vi "Read Analogue.vi"(8 "error in (no error)":errorcluster, 11 "Sim DMM in":refnum<class "Sim DMM.lvclass">) -> (0 "error out":errorcluster, 2 "Waveforms":waveform(dbl)[](array[waveform]), 3 "Sim DMM out":refnum<class "Sim DMM.lvclass">)   [LabVIEW 2025, in "DMM.lvlib" / "Sim DMM.lvclass"]
uses:
  Sim DMM.lvclass
  C:/Users/Public/Documents/Sandia National Labs/TSS Plugin/CEF.lvlibp/Node/CEF_Node.lvclass
  C:/Users/Public/Documents/Sandia National Labs/TSS Plugin/Abstract Engine.lvlibp/Abstract Instrument/Abstract Instrument.lvclass
  Users/Public/Documents/Sandia National Labs/TSS Plugin/Abstract Engine.lvlibp/Abstract Instrument/Channel.ctl
  DMM Channel/DMM Channel.lvclass
  Users/Public/Documents/Sandia National Labs/TSS Plugin/Abstract Engine.lvlibp/Channel configuration/Channel configuration.lvclass
  Users/Public/Documents/Sandia National Labs/TSS Plugin/CEF.lvlibp/Node/ReadChildren.vi
  Users/Public/Documents/Sandia National Labs/TSS Plugin/Abstract Engine.lvlibp/Channel configuration/Read Channel Setting.vi
  Users/Public/Documents/Sandia National Labs/TSS Plugin/CEF.lvlibp/Node/CEF_Node.lvclass
  Users/Public/Documents/Sandia National Labs/TSS Plugin/CEF.lvlibp/serializable configuration/CEF_serializable configuration.lvclass
  <vilib>/ptbypt/NI_PtbyPt.lvlib
  Users/Public/Documents/Sandia National Labs/TSS Plugin/Abstract Engine.lvlibp/Abstract Instrument/Abstract Instrument.lvclass
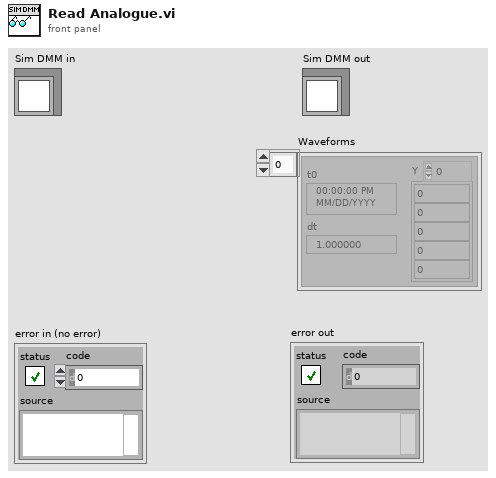
[diagram p1: front panel]
types:
  T1 = typedef "Abstract Engine.lvlibp/Abstract Instrument.lvclass/Channel.ctl" = cluster{"Alias":string, "DataType":enum16{"Anaolg Input", "Waveform"}, "Unit":enum16{"---", "V", "A", "Ohm", "Hz", "uF", "degC", "deg"}, "Upper limit":dbl, "Lower limit":dbl, "Measurement":variant}
  T2 = typedef "Abstract Engine.lvlibp/Channel configuration.lvclass/Default Channel.ctl" = cluster{"Address":string, "SW Alias":string, "Enabled":bool, "Type":string, "Description":string}
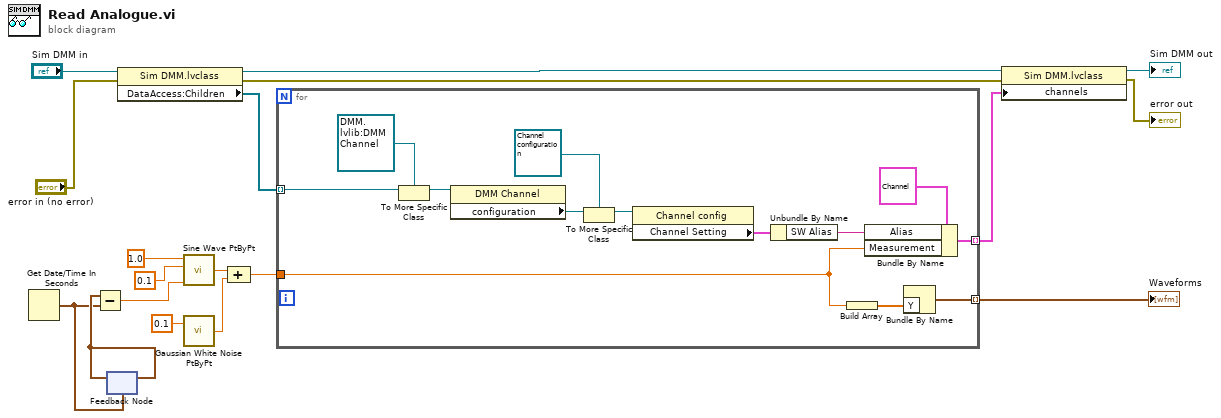
[diagram p0: block diagram]
diagram:
  n1 = Get Date/Time In Seconds() -> (seconds since 1Jan1904=w11:timestamp)
  n2 = feedback #1(w11) -> (w15:timestamp)
  n3 = Subtract(x=w15, y=w11) -> (x-y=w12:dbl)
  n4 = feedback-in #1(w15) -> ()
  n5 = property class="Sim DMM.lvclass"(reference="Sim DMM in", error in="error in (no error)") -> (reference out=w9:refnum<class "Sim DMM.lvclass">, error out=w4:errorcluster, "DataAccess:Children"=w8:refnum<data-value>[])
  n6 = call <vilib>:"Sine Wave PtByPt.vi"("time"=w12, "frequency"=0.1, "amplitude"=1.0) -> ("sine wave"=w17:dbl)  [unwired: 1 in]
  n7 = call <vilib>:"Gaussian White Noise PtByPt.vi"("standard deviation"=0.1) -> ("Gaussian white noise"=w16:dbl)  [unwired: 2 in]
  n8 = Compound Arithmetic op=ADD(w17, w16) -> (w7:dbl)
  n9 = for {
    tunnel: w8 -> [w31] mode=indexing
    tunnel: [w29] -> w2 mode=indexing
    tunnel: w7 -> [w27]
    tunnel: [w25] -> w1 mode=indexing
    n10 = To More Specific Class(target class=refnum<data-value> refnum ("data value reference"), reference=w31) -> (specific class reference=w24:refnum<data-value>)  [unwired: 1 in, 1 out]
    n11 = property class="DMM Channel"(reference=w24) -> ("configuration"=w23:refnum<class "CEF_serializable configuration.lvclass">)  [unwired: 1 in, 2 out]
    n12 = To More Specific Class(target class=refnum<class "Channel configuration.lvclass"> refnum ("Abstract Engine.lvlibp:Channel config"), reference=w23) -> (specific class reference=w22:refnum<class "Channel configuration.lvclass">)  [unwired: 1 in, 1 out]
    n13 = property class="Channel config"(reference=w22) -> ("Channel Setting"=w21:T2)  [unwired: 1 in, 2 out]
    n14 = Unbundle By Name(w21) -> ("SW Alias"=w30:string)
    n15 = Build Array(w27) -> (w26:dbl[])
    n16 = Bundle By Name(cluster=T1 {"Alias"="ch0", "DataType"=enum."Anaolg Input", "Unit"=enum."V", "Upper limit"=10.0, "Lower limit"=-10.0, "Measurement"=variant} ("Channel"), "Alias"=w30, "Measurement"=w27) -> (w29:T1)
    n17 = Bundle By Name("Y"=w26) -> (w25:waveform(dbl))  [unwired: 1 in]
  }
  "Waveforms" <- w1
  n18 = property class="Sim DMM.lvclass"(reference=w9, error in=w4, "channels"=w2) -> (reference out=→"Sim DMM out":refnum<class "Sim DMM.lvclass">, error out=→"error out":errorcluster)
